vi "MultiStation@ChangeState__Parameter.vi"(1 "ParamterIn":string) -> (0 "ParamterOut":string)   [LabVIEW 2020]
panel:
  in  "IDName":string(combo)
  in  "State":string(combo)
  in  "StationName":string(combo)
  in  "Confirm":bool
  # "MultiStation@ChangeState $Station.$ID,$State"
  # "."
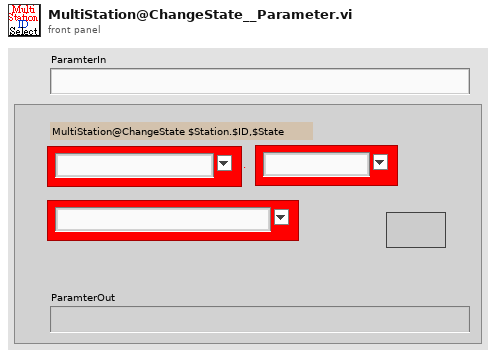
[diagram p1: front panel]
types:
  T1 = enum16{"Init", "AddStation", "StateShift", "ResetDefault", "SetStationON", "SetStationOFF", "SetStationOK", "SetStationNG", "UpdateIndicator", "SetData", "GetData", "GetOnOff", "GetOkNg", "ShowFeedInTray", "ShowFeedOutTray", "BlinkingOn", "BlinkingOff"}
  T2 = cluster{"轉盤燈號":refnum<vi>[], "各站資料":cluster{"轉盤燈號":bool, "錯誤燈號":bool, "資料":variant}[], "IDList":string[]}[]
  T3 = cluster{"轉盤燈號":refnum<vi>[], "各站資料":cluster{"轉盤燈號":bool, "錯誤燈號":bool, "資料":variant}[], "IDList":string[]}
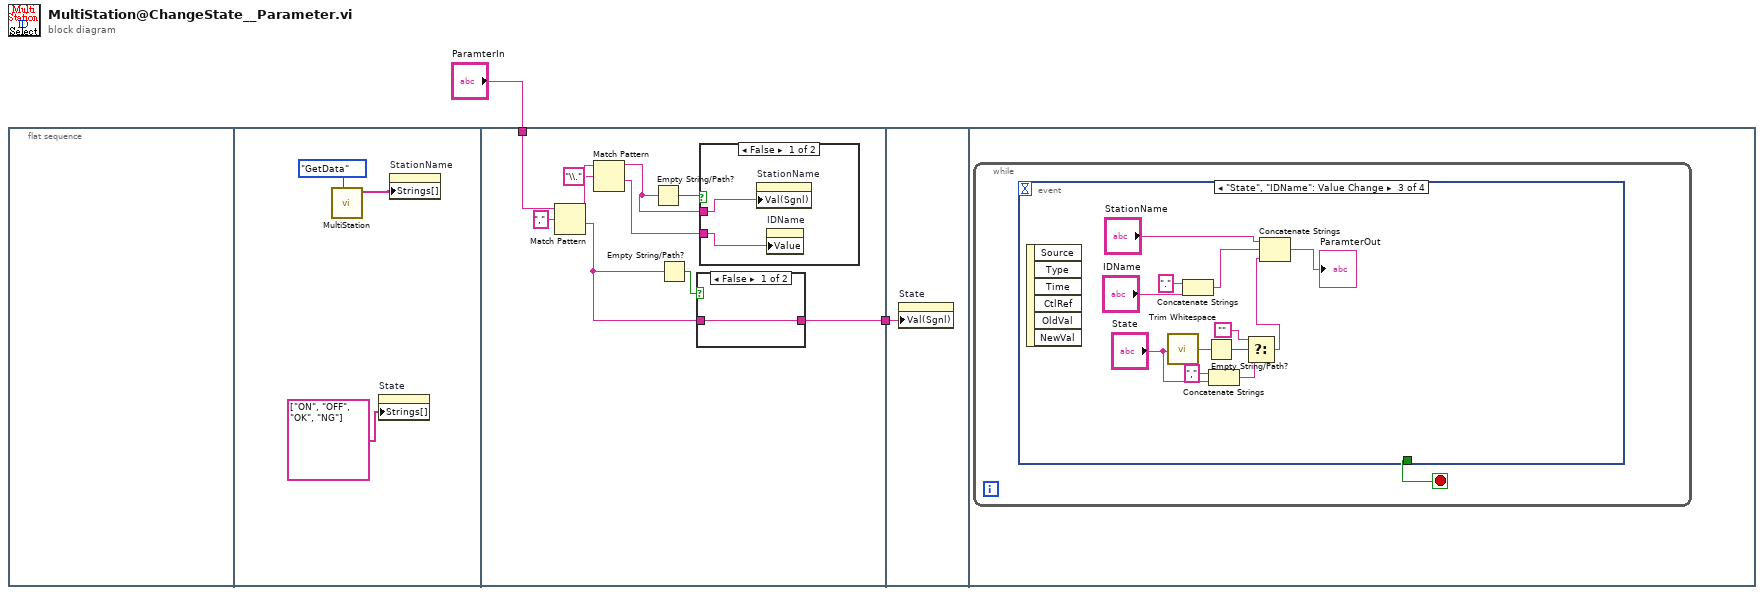
[diagram p0: block diagram]
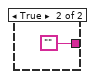
[diagram p2: hidden frame]
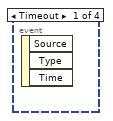
[diagram p4: hidden frame]
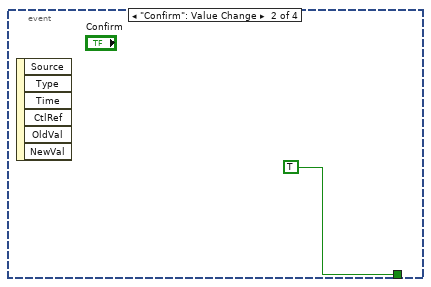
[diagram p5: hidden frame]
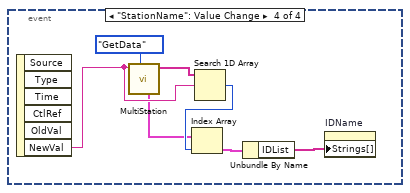
[diagram p6: hidden frame]
diagram:
  n1 = flat-sequence {
    tunnel: "ParamterIn" -> [w12]
    tunnel: [w13] -> w1
    tunnel: w1 -> [w20]
    frame #0 {
    }
    frame #1 {
      n2 = call "MultiStation.vi"("OP"=T1."GetData") -> ("StationList"=w4:string[])  [unwired: 6 in, 4 out]
      n3 = property on="State" class="CmbBox"("Strings[]"=string[] ["ON", "OFF", "OK", "NG"] ("Strings []")) -> ()  [unwired: 2 in, 2 out]
      n4 = property on="StationName" class="CmbBox"("Strings[]"=w4) -> ()  [unwired: 2 in, 2 out]
    }
    frame #2 {
      n5 = Match Pattern(string=w12, regular expression="," ("search string")) -> (before substring=w9:string, after substring=w10:string)  [unwired: 1 in, 2 out]
      n6 = Match Pattern(string=w9, regular expression="\\.") -> (before substring=w7:string, after substring=w6:string)  [unwired: 1 in, 2 out]
      n7 = Empty String/Path?(string/path=w7) -> (empty?=w15:bool)
      n8 = Empty String/Path?(string/path=w10) -> (empty?=w14:bool)
      n9 = case shown="False" w14 {
        tunnel: [w16 ""] -> w13
        tunnel: w10 -> [w16 _]
        frame False {
        }
        frame True {
        }
      }
      n10 = case shown="False" w15 {
        tunnel: w7 -> [w19 _]
        tunnel: w6 -> [w18 _]
        frame False {
          n11 = property on="StationName" class="CmbBox"("Val(Sgnl)"=w19) -> ()  [unwired: 2 in, 2 out]
          n12 = property on="IDName" class="CmbBox"("Value"=w18) -> ()  [unwired: 2 in, 2 out]
        }
        frame True {
        }
      }
    }
    frame #3 {
      n13 = property on="State" class="CmbBox"("Val(Sgnl)"=w20) -> ()  [unwired: 2 in, 2 out]
    }
    frame #4 {
      n14 = while {
        stop <- w21 stop-if-true
        n15 = event shown="[2] \"State\", \"IDName\": Value Change" {
          selector: _ -> [_ _ _ _]
          dyn-events: _ -> [_ _ _ _]
          timeout: _ -> [_ _ _ _]
          tunnel: [_ TRUE _ _] -> w21
          event Timeout {
            n16 = event-data() -> ()  [unwired: 1 in, 3 out]
          }
          event "Confirm": Value Change {
            n17 = event-data() -> ()  [unwired: 1 in, 6 out]
          }
          event "State", "IDName": Value Change {
            n18 = event-data() -> ()  [unwired: 1 in, 6 out]
            n19 = call <vilib>:"Trim Whitespace.vi"("string"="State") -> ("trimmed string"=w29:string)  [unwired: 1 in]
            n20 = Concatenate Strings("." ("string"), "IDName") -> (w23:string)
            n21 = Empty String/Path?(string/path=w29) -> (empty?=w30:bool)
            n22 = Concatenate Strings("," ("string"), "State") -> (w32:string)
            n23 = Select(t="", s=w30, f=w32) -> (s? t:f=w26:string)
            n24 = Concatenate Strings("StationName", w23, w26) -> (→"ParamterOut":string)
          }
          event "StationName": Value Change {
            n25 = event-data() -> ("NewVal"=w39:string)  [unwired: 1 in, 5 out]
            n26 = call "MultiStation.vi"("OP"=T1."GetData", "StationID"=w39) -> ("StationList"=w40:string[], "StationInfoS"=w37:T2)  [unwired: 5 in, 3 out]
            n27 = Search 1D Array(1D array=w40, element=w39) -> (index of element=w38:i32)  [unwired: 1 in]
            n28 = Index Array(array=w37, index=w38) -> (element=w36:T3)
            n29 = Unbundle By Name(w36) -> ("IDList"=w35:string[])
            n30 = property on="IDName" class="CmbBox"("Strings[]"=w35) -> ()  [unwired: 2 in, 2 out]
          }
        }
      }
    }
  }
